vi "Save TabAcqType index.vi"(8 "error in (no error)":errorcluster, 11 "S4GUI in":refnum<class "S4GUI.lvclass">) -> (0 "error out":errorcluster, 3 "S4GUI out":refnum<class "S4GUI.lvclass">)   [LabVIEW 2018, in "S4GUI.lvclass"]
uses:
  S4GUI.lvclass
  S4GUI.lvclass/S4GUI.ctl
  <vilib>/Utility/config.llb/Write Key (U32).vi
  <vilib>/Utility/config.llb/NI_LVConfig.lvlib
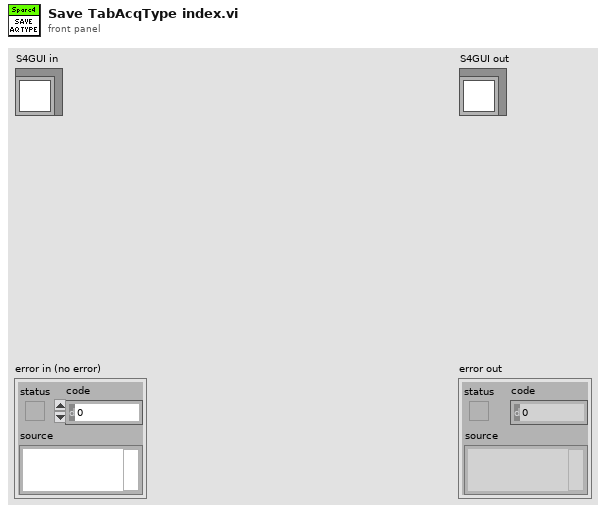
[diagram p1: front panel]
types:
  T1 = typedef "NI_LVConfig.lvlib/Config Data RefNum.ctl" = refnum<k1>
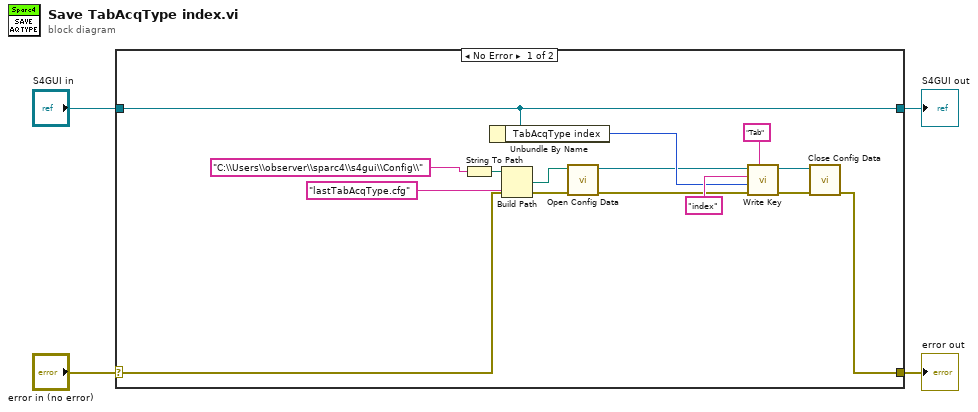
[diagram p0: block diagram]
diagram:
  n1 = case shown="No Error" "error in (no error)" {
    selector: "error in (no error)" -> [w6 w20]
    tunnel: [w5 w20] -> w3
    tunnel: [w10 w19] -> w1
    tunnel: "S4GUI in" -> [w10 w19]
    frame No Error {
      n2 = String To Path(string="C:\\Users\\observer\\sparc4\\s4gui\\Config\\") -> (path=w17:path)
      n3 = Unbundle By Name(w10) -> ("TabAcqType index"=w9:u32)
      n4 = Build Path(base path=w17, name or relative path="lastTabAcqType.cfg") -> (appended path=w18:path)
      n5 = call <vilib>:"Open Config Data.vi"("error in (no error)"=w6, "configuration file path"=w18) -> ("error out"=w7:errorcluster, "refnum"=w8:T1)  [unwired: 7 in, 1 out]
      n6 = call-poly <vilib>:"Write Key.vi"("section"="Tab", "error in (no error)"=w7, "value"=w9, "key"="index", "refnum"=w8) -> ("error out"=w12:errorcluster, "refnum out"=w13:T1)  [unwired: 4 in, 1 out]
      n7 = call <vilib>:"Close Config Data.vi"("error in (no error)"=w12, "refnum"=w13) -> ("error out"=w5:errorcluster)  [unwired: 8 in, 1 out]
    }
    frame Error {
    }
  }
  "error out" <- w3
  "S4GUI out" <- w1
